vi "Set and Get Active Row Cell Justify and Height.vi"(6 "Active Row":i32, 7 "Mode":T1, 8 "错误输入":errorcluster, 9 "Cell Height In":i32, 10 "Justify In":enum16{"Left", "Center", "Right"}(ring), 11 "Listbox Ref":refnum<vi>) -> (0 "错误输出":errorcluster, 1 "Cell Height":i32, 2 "Justify":enum16{"Left", "Center", "Right"}(ring), 3 "Dup Listbox Ref":refnum<vi>)   [LabVIEW 2011, in "Listbox Tool.lvlib"]
uses:
  Listbox Tool.lvlib
  Custom Type/Read and Write Mode.ctl
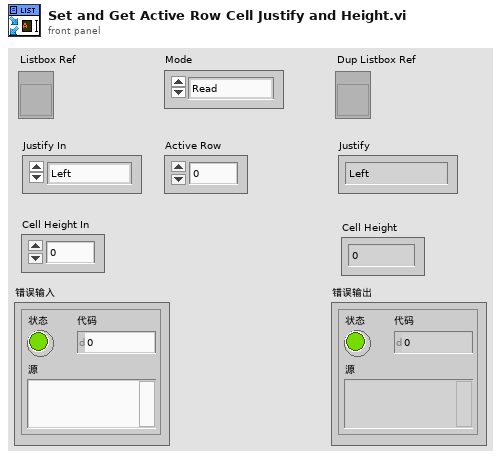
[diagram p1: front panel]
types:
  T1 = typedef "Listbox Tool.lvlib/Read and Write Mode.ctl" = enum16{"Read", "Write"}
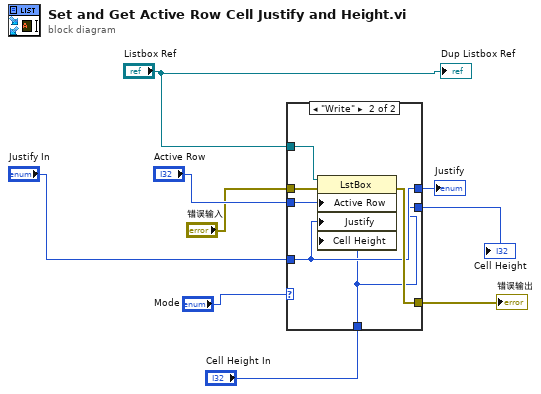
[diagram p0: block diagram]
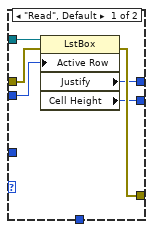
[diagram p2: hidden frame]
diagram:
  n1 = case shown="\"Write\"" "Mode" {
    tunnel: "Listbox Ref" -> [w14 w19]
    tunnel: "Active Row" -> [w12 w21]
    tunnel: "错误输入" -> [w15 w20]
    tunnel: [w13 w18] -> w6
    tunnel: "Justify In" -> [_ w17]
    tunnel: "Cell Height In" -> [_ w16]
    tunnel: [w11 w17] -> w4
    tunnel: [w10 w16] -> w3
    frame "Read", Default {
      n2 = property class="LstBox"(reference=w14, error in=w15, "Active Row"=w12) -> (error out=w13:errorcluster, "Justify"=w11:enum16{"Left", "Center", "Right"}, "Cell Height"=w10:i32)  [unwired: 1 out]
    }
    frame "Write" {
      n3 = property class="LstBox"(reference=w19, error in=w20, "Active Row"=w21, "Justify"=w17, "Cell Height"=w16) -> (error out=w18:errorcluster)  [unwired: 1 out]
    }
  }
  "错误输出" <- w6
  "Justify" <- w4
  "Cell Height" <- w3
  "Dup Listbox Ref" <- "Listbox Ref"
